vi "Down Casting Example.vi"() -> ()   [LabVIEW 2017]
uses:
  Event Data Types/Event Boolean/Event Boolean.lvclass
  C:/Projects/Shared Libraries/Event Actors/Event/Event.lvclass
  Event/Event.lvclass
panel:
  out "specific class reference":refnum<class "Event Boolean.lvclass">
  out "error out":errorcluster
  in  "error in":errorcluster
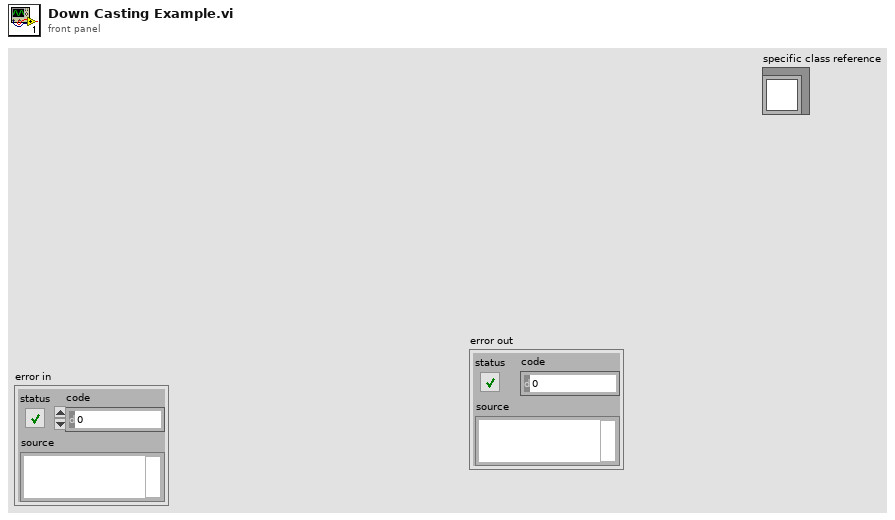
[diagram p1: front panel]
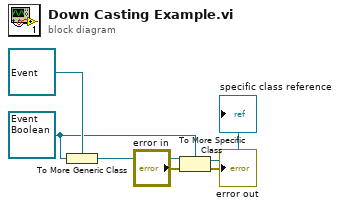
[diagram p0: block diagram]
diagram:
  w2 = refnum<class "Event Boolean.lvclass"> refnum ("Event Actors.lvlib:Event Boolean.lvclass")
  n1 = To More Generic Class(target class=refnum<class "Event.lvclass"> refnum ("Event Actors.lvlib:Event"), reference=w2) -> (generic class reference=w5:refnum<class "Event.lvclass">)
  n2 = To More Specific Class(target class=w2, reference=w5, error in="error in") -> (specific class reference=→"specific class reference":refnum<class "Event Boolean.lvclass">, error out=→"error out":errorcluster)
